vi "SeCrTs-AO_Element to WF.vi"(11 "AO Array":dbl) -> (3 "Array":waveform(dbl)[](array[waveform]))   [LabVIEW 2022 SP3]
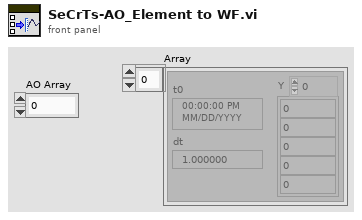
[diagram p1: front panel]
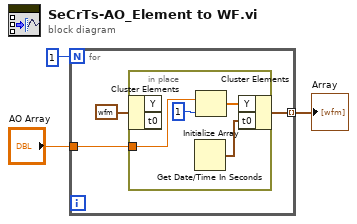
[diagram p0: block diagram]
diagram:
  n1 = for {
    N: 1 -> [_]
    tunnel: "AO Array" -> [w6]
    tunnel: [w5] -> w3 mode=indexing
    n2 = in-place {
      in-place-border: w6 -> [w8]
      n3 = in-place-cluster #1(waveform(dbl) {"t0"=timestamp(0 s since 1904-01-01), "dt"=0.001, "Y"=[]} ("waveform")) -> ()  [unwired: 2 out]
      n4 = Get Date/Time In Seconds() -> (seconds since 1Jan1904=w10:timestamp)
      n5 = Initialize Array(w8, 1 ("dimension size")) -> (w7:dbl[])
      n6 = in-place-cluster #1("Y"=w7, "t0"=w10) -> (w5:waveform(dbl))
    }
  }
  "Array" <- w3
